vi "NISE.remote.Build URL.vi"(7 "https?":bool, 9 "Port":u16, 10 "Hostname/IP":string, 11 "service name":string) -> (2 "URL":string)   [LabVIEW 2016, in "SLSC Interface.lvclass"]
uses:
  SLSC Interface Class/SLSC Interface.lvclass
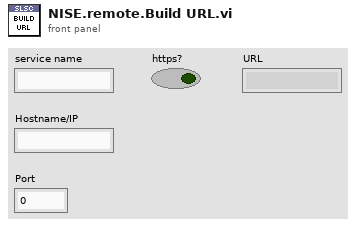
[diagram p1: front panel]
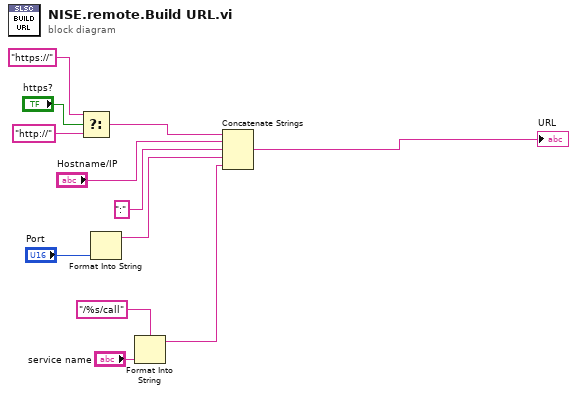
[diagram p0: block diagram]
diagram:
  n1 = Select(t="https://" ("Hostname/IP"), s="https?", f="http://") -> (s? t:f=w8:string)
  n2 = Format Into String("Port") -> (resulting string=w11:string)  [unwired: 3 in, 1 out]
  n3 = Format Into String(format string="/%s/call", "service name") -> (resulting string=w2:string)  [unwired: 2 in, 1 out]
  n4 = Concatenate Strings(w8, "Hostname/IP", ":" ("string"), w11, w2) -> (→"URL":string)
